vi "Write SlotTime(ms).vi"(8 "error in (no error)":errorcluster, 10 "SlotTime(ms)":u32, 11 "FrameSlot_Root in":refnum<class "FrameSlot_Root.lvclass">) -> (0 "error out":errorcluster, 3 "FrameSlot_Root out":refnum<class "FrameSlot_Root.lvclass">)   [LabVIEW 2018, in "FrameSlot_Root.lvclass"]
uses:
  FrameSlot_Root.lvclass
  FrameSlot_Root.lvclass/FrameSlot_Root.ctl
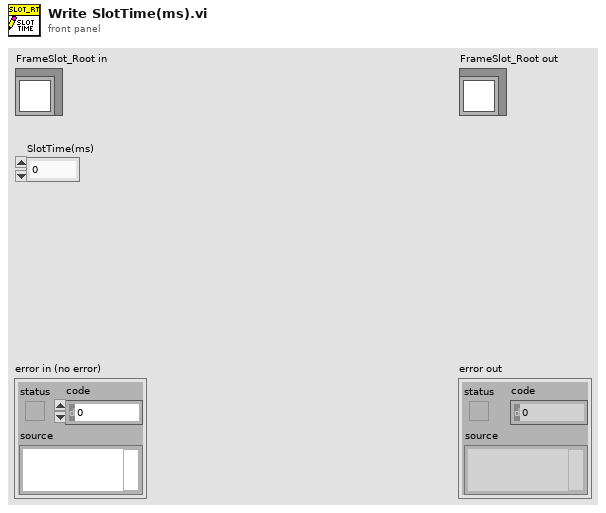
[diagram p1: front panel]
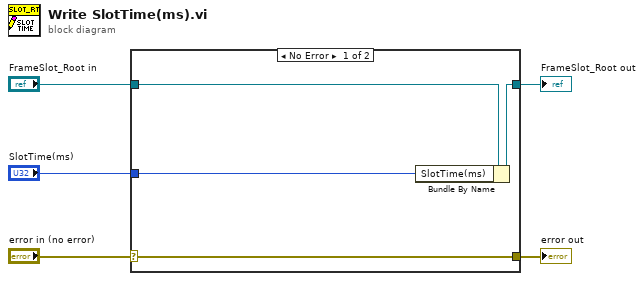
[diagram p0: block diagram]
diagram:
  n1 = case shown="No Error" "error in (no error)" {
    selector: "error in (no error)" -> [w9 w10]
    tunnel: [w9 w10] -> w4
    tunnel: [w7 w11] -> w2
    tunnel: "FrameSlot_Root in" -> [w8 w11]
    tunnel: "SlotTime(ms)" -> [w6 _]
    frame No Error {
      n2 = Bundle By Name(cluster=w8, "SlotTime(ms)"=w6) -> (w7:refnum<class "FrameSlot_Root.lvclass">)
    }
    frame Error {
    }
  }
  "error out" <- w4
  "FrameSlot_Root out" <- w2
